vi "Write File Ref.vi"(8 "error in (no error)":errorcluster, 10 "File Ref":refnum<k34>, 11 "Error Logger in":refnum<class "Error Logger.lvclass">) -> (0 "error out":errorcluster, 3 "Error Logger out":refnum<class "Error Logger.lvclass">)   [LabVIEW 2012, in "Error Logger.lvclass"]
uses:
  Error Logger.lvclass
  Error Logger.lvclass/Error Logger.ctl
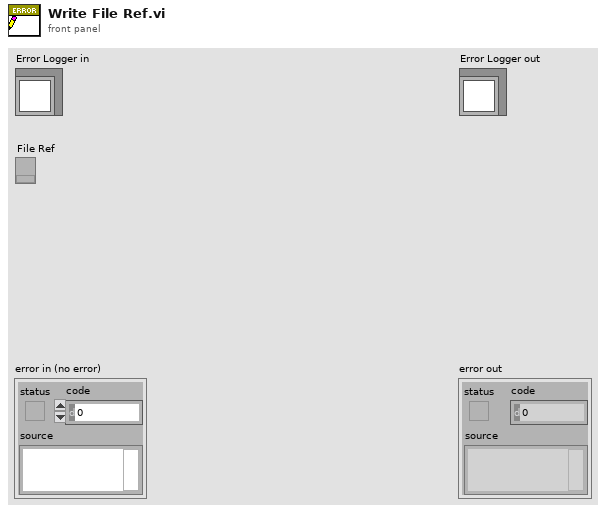
[diagram p1: front panel]
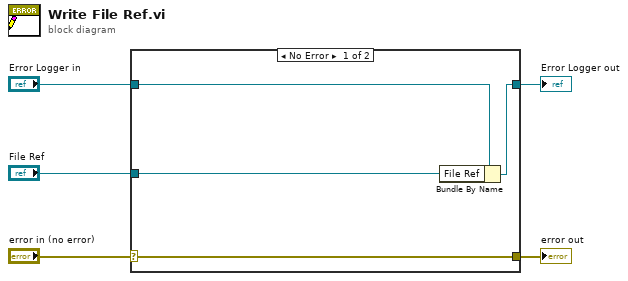
[diagram p0: block diagram]
diagram:
  n1 = case shown="No Error" "error in (no error)" {
    selector: "error in (no error)" -> [w9 w10]
    tunnel: [w9 w10] -> w4
    tunnel: [w7 w11] -> w2
    tunnel: "Error Logger in" -> [w8 w11]
    tunnel: "File Ref" -> [w6 _]
    frame No Error {
      n2 = Bundle By Name(cluster=w8, "File Ref"=w6) -> (w7:refnum<class "Error Logger.lvclass">)
    }
    frame Error {
    }
  }
  "error out" <- w4
  "Error Logger out" <- w2
